vi "Scale.vi"(8 "error in (no error)":errorcluster, 10 "Scale Factor":dbl, 11 "Triangle in":refnum<class "Losange.lvclass">) -> (0 "error out":errorcluster, 3 "Triangle out":refnum<class "Losange.lvclass">)   [LabVIEW 2021, in "Picture2D.lvlib" / "Losange.lvclass"]
uses:
  Losange.lvclass
  Polygone/Polygone.lvclass
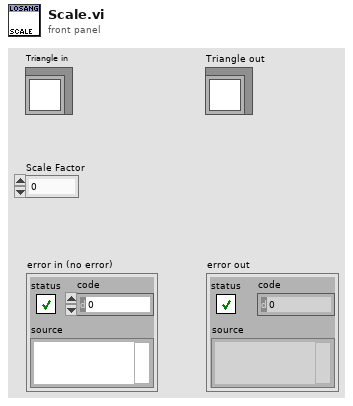
[diagram p1: front panel]
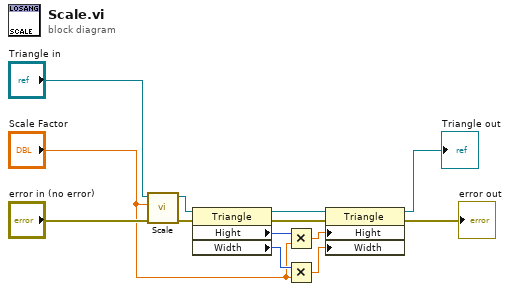
[diagram p0: block diagram]
diagram:
  n1 = call-parent "Scale.vi"("error in (no error)"="error in (no error)", "Scale Factor"="Scale Factor", "Shape in"="Triangle in") -> ("error out"=w3:errorcluster, "Shape out"=w11:refnum<class "Losange.lvclass">)  [unwired: 7 in]
  n2 = property class="Triangle"(reference=w11, error in=w3) -> (reference out=w4:refnum<class "Losange.lvclass">, error out=w2:errorcluster, "Hight"=w9:i16, "Width"=w7:i16)
  n3 = Multiply(x=w9, y="Scale Factor") -> (x*y=w8:dbl)
  n4 = Multiply(x=w7, y="Scale Factor") -> (x*y=w6:dbl)
  n5 = property class="Triangle"(reference=w4, error in=w2, "Hight"=w8, "Width"=w6) -> (reference out=→"Triangle out":refnum<class "Losange.lvclass">, error out=→"error out":errorcluster)
